vi "Simulated Mecanum Robot.vi"() -> ()   [LabVIEW 2017]
doc: "This example demonstrates the control of an autonomous robot through multiple asynchronous processes, modeled by VIs, that communicate with each other using shared variables. This example also shows an obstacle avoidance algorithm that the simulated robot uses as it navigates. The application includes the following processes:\n\n1. LIDAR Loop (\"Sense\")--Uses LabVIEW dataflow programming to generate simulated sensor data based on the position of the robot and any obstacles in the environment.\n\n2. Operator Loop (\"Think\")--Uses a state machine to control the movement of the robot according to commands from the user. When the robot follows a path without joystick or keyboard control, this process controls the attitude of the autonomous robot using a Vector Field Histogram (VFH) algorithm to avoid obstacles.\n\n3. Motor Loop (\"Act\")--Uses a Control and Simulation Loop, from the Control Design and Simulation Module, to create a model of the robot, simulate its dynamic behavior, and show the control loops and attitude observers."
uses:
  <vilib>/Utility/miscctls.llb/LVPointTypeDef.ctl
  <vilib>/Platform/TimedLoop/XDataNode/timing_clust.ctl
  <vilib>/Platform/TimedLoop/XDataNode/nitl_modes.ctl
  <vilib>/Platform/TimedLoop/XDataNode/wakeup.ctl
  <vilib>/Utility/miscctls.llb/LV3DPointTypeDef.ctl
  <vilib>/Platform/TimedLoop/XDataNode/XDataNode.xnode
  <vilib>/Platform/TimedLoop/XDataNode/XDNodeRunTimeDep.lvlib
panel:
  in  "Show LL Diagram":bool
  in  "Show OL Diagram":bool
  in  "Show MCL Diagram":bool
  out "RR Wheel N":dbl(slide)
  out "RR Wheel":dbl(slide) scale=0.0..15.0
  out "RL Wheel N":dbl(slide)
  out "RL Wheel":dbl(slide) scale=0.0..15.0
  out "FL Wheel N":dbl(slide)
  out "FL Wheel":dbl(slide) scale=0.0..15.0
  out "FR Wheel N":dbl(slide)
  out "FR Wheel":dbl(slide) scale=0.0..15.0
  in  "Rotate Left":dbl(slide) scale=0.0..1.0
  in  "Rotate Right":dbl(slide) scale=0.0..1.0
  in  "Left":dbl(slide)
  in  "Right":dbl(slide) scale=0.0..1.0
  in  "Backward":dbl(slide)
  in  "Forward":dbl(slide) scale=0.0..1.0
  in  "Camera Control":enum32{"Free", "Observer View", "Robot View"}(radio)
  in  "About":bool
  in  "Robot Mode:":enum16{"Idle", "Tele-Op", "Path Following"}(ring)=enum."Tele-Op"
  in  "VFH Visualization":bool
  out "Obstacle Map":picture
  out "End Loop":bool=TRUE
  in  "Stop":bool
  out "3D Visualization":refnum<vi>(3d-picture)
  # "Instructions:\n\n1. If you want to use a joystick to control the simulated robot, install the joystick before you run this VI.\n\n2. Run VI.  Click the About This Example button for more information about the simulated robot.\n\n3. Use the joystick or press keypad buttons to move the robot.\n\n4. Click a position in the Obstacle Map to change the target position of the robot.\n\n5. Click the Robot Mode control and select Path Following to command the robot to navigate to the target based on vector field histogram data about the environment.\n\n6. Click the VFH Visualization button to launch the VFH Visualization VI, in which you can observe the vector field histogram data.\n\n7. Click the buttons in the VI Block Diagram Visualization section to view the code that controls the robot.  You also can press the <Ctrl-E> keys to view the block diagram of the main VI."
  # "VI Block Diagram Visualization"
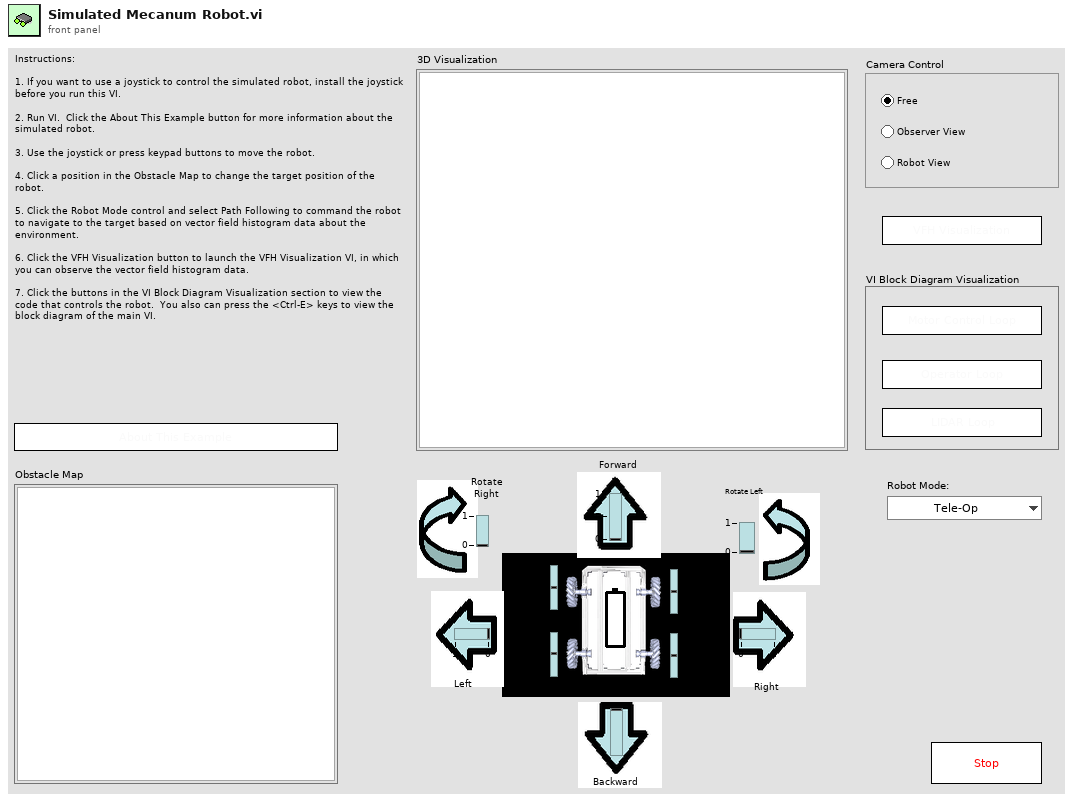
[diagram p1: front panel]
types:
  T1 = typedef "LVPointTypeDef.ctl" = cluster{"Horizontal":i16, "Vertical":i16}
  T2 = typedef "LVBoundsTypeDef.ctl" = cluster{"Width":u32, "Height":u32}
  T3 = typedef "XDNodeRunTimeDep.lvlib/timing_clust.ctl" = cluster{"Expected End [f-1]":u64, "Actual End [f-1]":u64, "Finished Late? [f-1]":bool, "Expected End [i-1]":u64, "Actual End [i-1]":u64, "Finished Late? [i-1]":bool, "Expected Start [i]":u64, "Actual Start [i]":u64, "Expected Start [f]":u64, "Actual Start [f]":u64, "Source Name":string, "Structure Name":string, "Period":i64, "Deadline":i64, "Offset":i64, "Start":i64, "Priority":i32, "Timeout":i32, "Mode":T4, "Wakeup Reason":T5, "Error":errorcluster, "Source Type":string, "Secondary Source Type":string, "Global End Time":u64, "Global Start Time":u64, "Frame Duration":u64, "Iteration Duration":u64, "Assigned CPU":i32, "I/O Scan Engine Mode":u32}
  T4 = typedef "XDNodeRunTimeDep.lvlib/nitl_modes.ctl" = enum32{"No Change", "Process missed periods, maintain original phase", "Discard missed periods, maintain original phase", "Process missed periods, ignore original phase", "Discard missed periods, ignore original phase"}
  T5 = typedef "XDNodeRunTimeDep.lvlib/wakeup.ctl" = enum32{"Normal", "Aborted", "Asynchronous wakeup", "Timing source error", "Timed loop error", "Timeout"}
  T6 = typedef "LVPoint32TypeDef.ctl" = cluster{"Horizontal":i32, "Vertical":i32}
  T7 = typedef "eventvkey.ctl" = enum16{"ASCII", "Enter", "Return", "Shift", "Ctrl", "Alt", "Cmd", "Opt", "Caps", "NumLock", "Clear", "Break", "Up", "Down", "Left", "Right", "Insert", "Delete", "Home", "End", "PageUp", "PageDown", "Escape", "Help", "Pause", "ScrollLock", "F1", "F2", "F3", "F4", "F5", "F6", "F7", "F8", "F9", "F10", "F11", "F12", "F13", "F14", "F15", "F16", "F17", "F18", "F19", "F20", "F21", "F22", "F23", "F24", "Play", "VolumeUp", "VolumeDown", "Mute", "Two Byte Char"}
  T8 = enum16{"Ignore", "Left", "Right", "Up", "Down", "CL", "CC"}
  T9 = typedef "LV3DPointTypeDef.ctl" = cluster{"X":sgl, "Y":sgl, "Z":sgl}
  T10 = cluster{"Array of Double[0]":dbl, "Array of Double[1]":dbl}
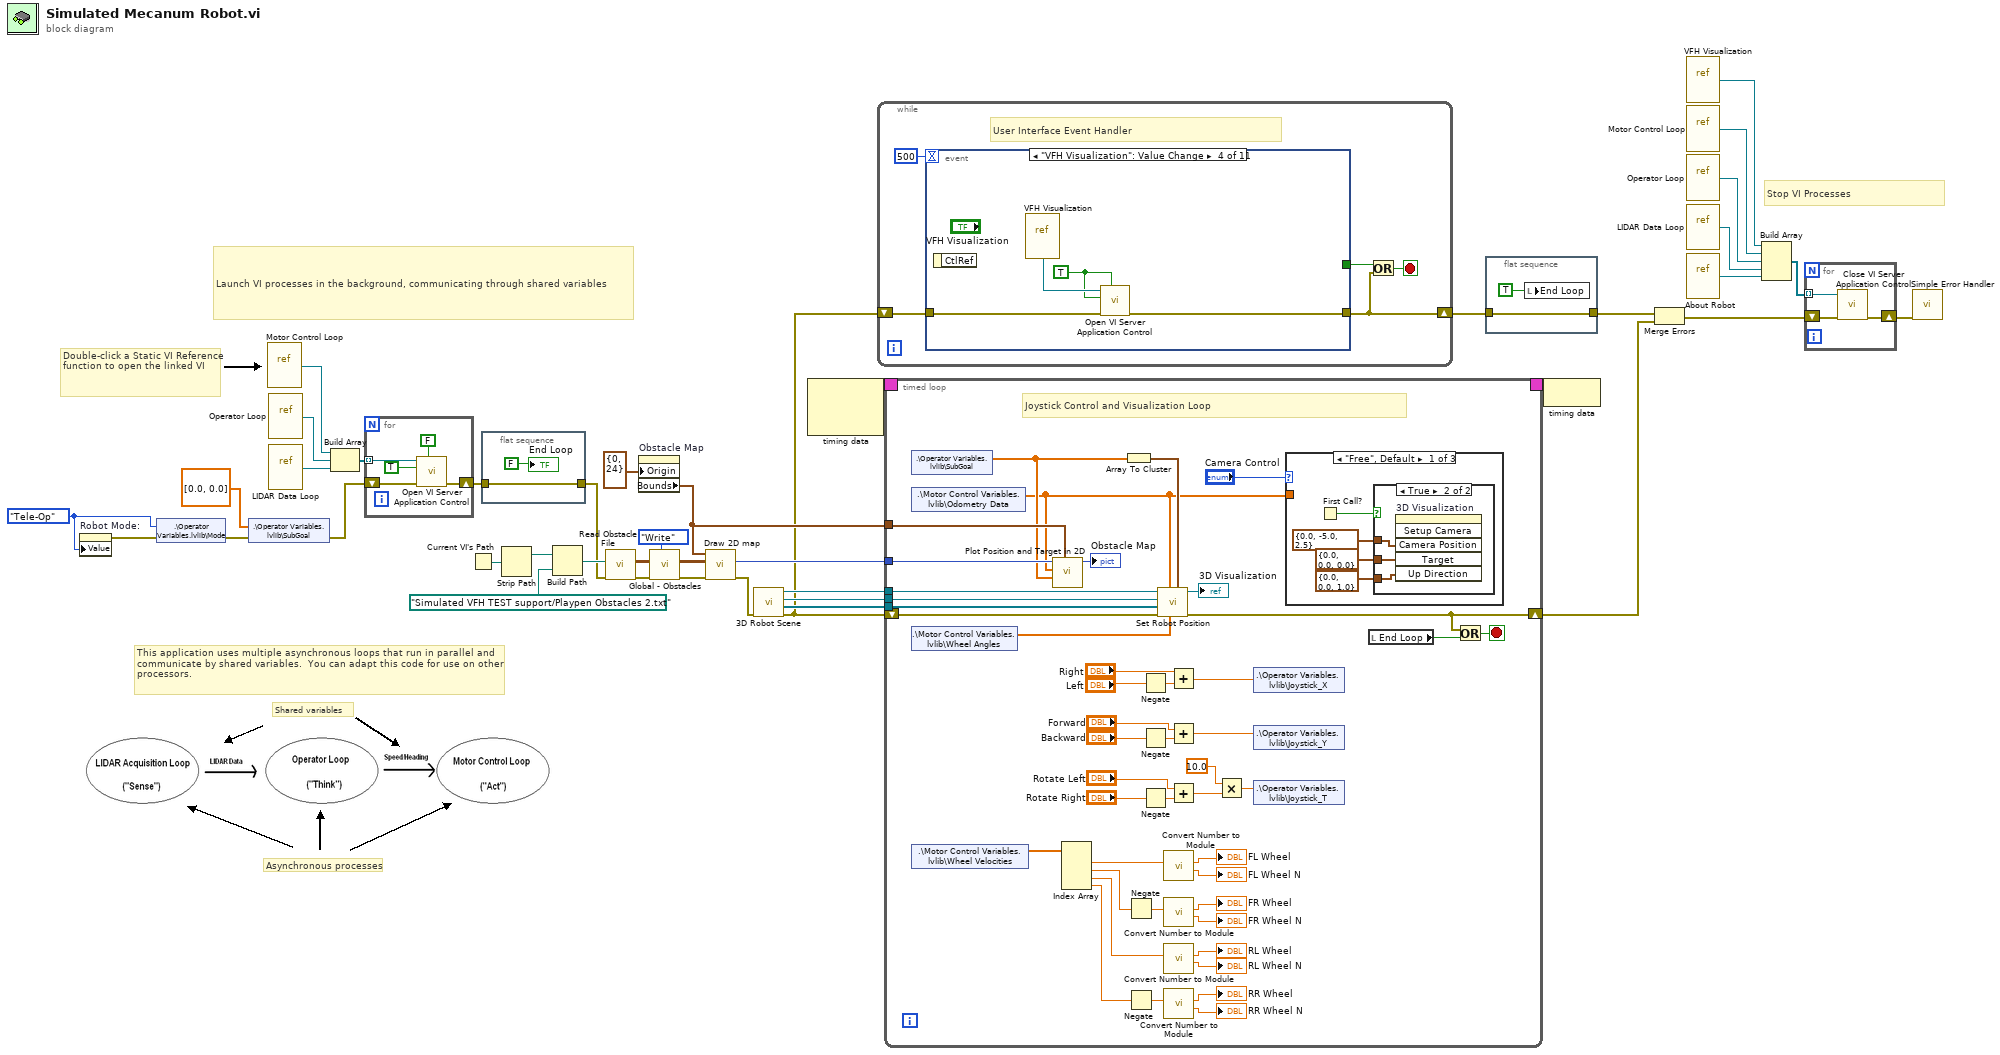
[diagram p0: block diagram]
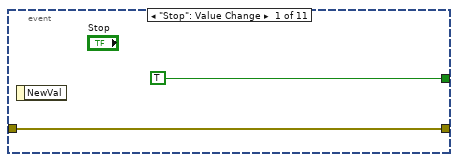
[diagram p2: hidden frame]
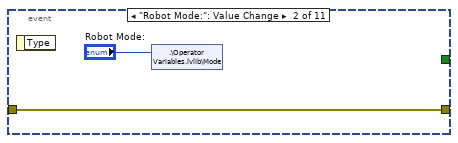
[diagram p3: hidden frame]
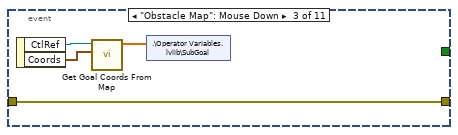
[diagram p4: hidden frame]
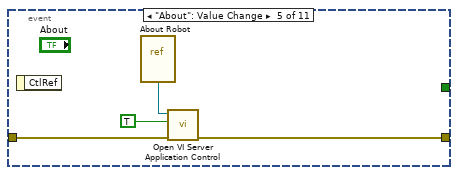
[diagram p5: hidden frame]
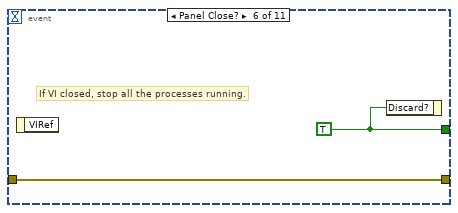
[diagram p6: hidden frame]
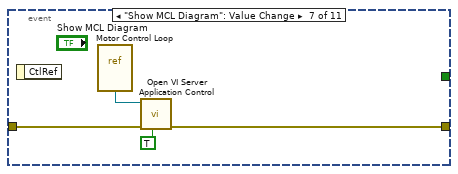
[diagram p7: hidden frame]
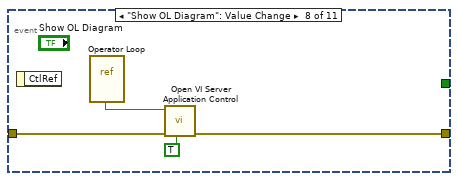
[diagram p8: hidden frame]
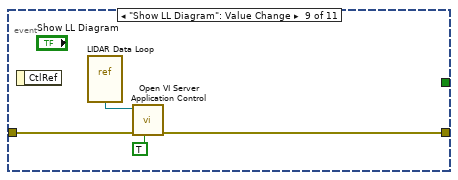
[diagram p9: hidden frame]
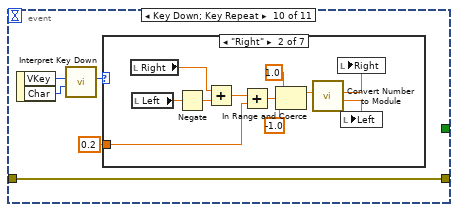
[diagram p10: hidden frame]
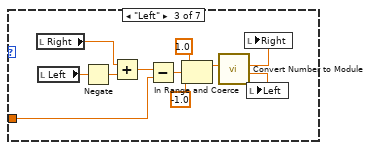
[diagram p12: hidden frame]
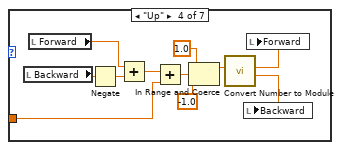
[diagram p13: hidden frame]
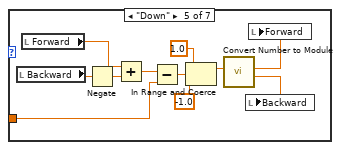
[diagram p14: hidden frame]
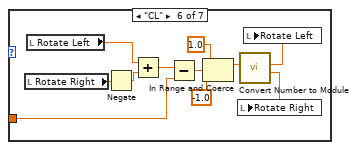
[diagram p15: hidden frame]
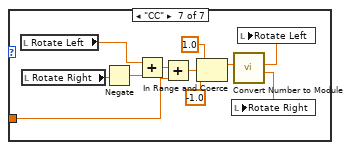
[diagram p16: hidden frame]
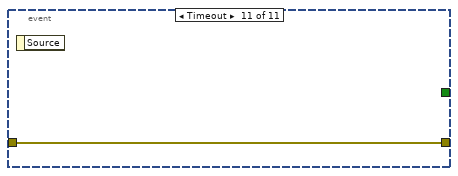
[diagram p17: hidden frame]
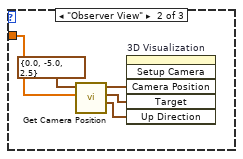
[diagram p19: hidden frame]
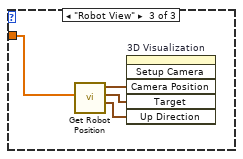
[diagram p20: hidden frame]
diagram:
  w8 = enum16{"Idle", "Tele-Op", "Path Following"}."Tele-Op" ("Mode")
  # "Launch VI processes in the background, communicating through shared variables"
  # "Stop VI Processes"
  # "Shared variables"
  # "Asynchronous processes"
  # "This application uses multiple asynchronous loops that run in parallel and communicate by shared variables.  You can adapt this code for use on other processors."
  # "Double-click a Static VI Reference function to open the linked VI"
  n1 = property on="Robot Mode:" class="Enum (strict)"("Value"=w8) -> (error out=w9:errorcluster)  [unwired: 2 in, 1 out]
  n2 = shared-variable ".\\Operator Variables.lvlib\\Mode"(w8, error in=w9) -> (error out=w4:errorcluster)
  n3 = shared-variable ".\\Operator Variables.lvlib\\SubGoal"(dbl[] [0.0, 0.0] ("SubGoal"), error in=w4) -> (error out=w3:errorcluster)
  n4 = vi-ref "Motor Control Loop.vi"() -> (w26:refnum<vi>)
  n5 = vi-ref "Operator Loop.vi"() -> (w23:refnum<vi>)
  n6 = vi-ref "LIDAR Data Loop.vi"() -> (w22:refnum<vi>)
  n7 = Build Array(w26, w23, w22) -> (w25:refnum<vi>[])
  n8 = for {
    tunnel: w25 -> [w46] mode=indexing
    shift-right: [w43] -> w7
    shift-left: w3 -> [w42]
    n9 = call "Open VI Server Application Control.vi"("open front panel (F)"=FALSE ("Open Front Panel"), "error in (no error)"=w42, "run VI (F)"=TRUE ("Run VI"), "VI refnum"=w46) -> ("error out"=w43:errorcluster)  [unwired: 7 in]
  }
  n10 = Current VI's Path() -> (path=w33:path)
  n11 = flat-sequence {
    tunnel: w7 -> [w48]
    tunnel: [w48] -> w6
    frame #0 {
      "End Loop" <- FALSE ("Halt TL")
    }
  }
  n12 = Strip Path(path=w33) -> (stripped path=w29:path)  [unwired: 1 out]
  n13 = Build Path(base path=w29, name or relative path=path "Simulated VFH TEST support/Playpen Obstacles 2.txt" ("file path for obstacle data")) -> (appended path=w32:path)
  n14 = call "Read Obstacle File.vi"("error in (no error)"=w6, "file path (use dialog)"=w32) -> ("error out"=w34:errorcluster, "obstacles (n x 2 array of pts)"=w35:cluster{dbl, dbl}[][])  [unwired: 8 in]
  n15 = property on="Obstacle Map" class="Pict"("Origin"=T1 {"Horizontal"=0, "Vertical"=24}) -> ("Bounds"=w37:T2)  [unwired: 2 in, 2 out]
  n16 = call "Global - Obstacles.vi"("mode"=enum16{"Initialize", "Read", "Write"}."Write" ("Mode"), "error in (no error)"=w34, "obstacles in"=w35) -> ("error out"=w30:errorcluster, "obstacles out"=w31:cluster{dbl, dbl}[][])  [unwired: 6 in, 1 out]
  n17 = call "Draw 2D map.vi"("error in (no error)"=w30, "obstacles"=w31, "bounds"=w37) -> ("error out"=w24:errorcluster, "picture"=w38:picture)  [unwired: 7 in]
  n18 = call "3D Robot Scene.vi"("error in (no error)"=w24) -> ("error out"=w5:errorcluster, "axles"=w41:refnum<vi>[], "robot"=w40:refnum<vi>, "scene"=w39:refnum<vi>)  [unwired: 7 in]
  n19 = node-c288() -> (w28:T3)  [unwired: 2 in]
  n20 = while {
    shift-right: [w49] -> w13
    shift-left: w5 -> [w53]
    stop <- w52 stop-if-true
    # "User Interface Event Handler"
    n21 = event shown="[3] \"VFH Visualization\": Value Change" {
      selector: _ -> [_ _ _ _ _ _ _ _ _ _ _]
      dyn-events: _ -> [_ _ _ _ _ _ _ _ _ _ _]
      timeout: 500 -> [_ _ _ _ _ _ _ _ _ _ _]
      tunnel: [TRUE _ _ _ _ w70 _ _ _ _ _] -> w51
      tunnel: w53 -> [w55 w56 w58 w63 w68 w71 w73 w77 w81 w84 w155]
      tunnel: [w55 w56 w58 w62 w67 w71 w72 w76 w80 w84 w155] -> w49
      event "Stop": Value Change {
        n22 = event-data() -> ()  [unwired: 2 out]
      }
      event "Robot Mode:": Value Change {
        n23 = event-data() -> ()  [unwired: 2 out]
        n24 = shared-variable ".\\Operator Variables.lvlib\\Mode"("Robot Mode:") -> ()  [unwired: 1 in, 1 out]
      }
      event "Obstacle Map": Mouse Down {
        n25 = event-data() -> ("CtlRef"=w60:refnum<vi>, "Coords"=w59:T6)  [unwired: 1 out]
        n26 = call "Get Goal Coords From Map.vi"("Coords"=w59, "CtlRef"=w60) -> ("Goal Coords"=w61:dbl[])  [unwired: 9 in]
        n27 = shared-variable ".\\Operator Variables.lvlib\\SubGoal"(w61) -> ()  [unwired: 1 in, 1 out]
      }
      event "VFH Visualization": Value Change {
        w64 = TRUE ("Launch Map")
        n28 = event-data() -> ()  [unwired: 2 out]
        n29 = vi-ref "VFH Visualization.vi"() -> (w65:refnum<vi>)
        n30 = call "Open VI Server Application Control.vi"("open front panel (F)"=w64, "error in (no error)"=w63, "run VI (F)"=w64, "VI refnum"=w65) -> ("error out"=w62:errorcluster)  [unwired: 7 in]
      }
      event "About": Value Change {
        n31 = event-data() -> ()  [unwired: 2 out]
        n32 = vi-ref "About Robot.vi"() -> (w69:refnum<vi>)
        n33 = call "Open VI Server Application Control.vi"("error in (no error)"=w68, "run VI (F)"=TRUE ("Launch Map"), "VI refnum"=w69) -> ("error out"=w67:errorcluster)  [unwired: 8 in]
      }
      event Panel Close? {
        w70 = TRUE ("Discard?")
        # "If VI closed, stop all the processes running."
        n34 = event-data() -> ()  [unwired: 2 out]
        n35 = event-data("Discard?"=w70) -> ()  [unwired: 1 in, 1 out]
      }
      event "Show MCL Diagram": Value Change {
        n36 = event-data() -> ()  [unwired: 2 out]
        n37 = vi-ref "Motor Control Loop.vi"() -> (w75:refnum<vi>)
        n38 = call "Open VI Server Application Control.vi"("open block diagram (F)"=TRUE ("Open Front Panel"), "error in (no error)"=w73, "VI refnum"=w75) -> ("error out"=w72:errorcluster)  [unwired: 8 in]
      }
      event "Show OL Diagram": Value Change {
        n39 = event-data() -> ()  [unwired: 2 out]
        n40 = vi-ref "Operator Loop.vi"() -> (w78:refnum<vi>)
        n41 = call "Open VI Server Application Control.vi"("open block diagram (F)"=TRUE ("Open Front Panel"), "error in (no error)"=w77, "VI refnum"=w78) -> ("error out"=w76:errorcluster)  [unwired: 8 in]
      }
      event "Show LL Diagram": Value Change {
        n42 = event-data() -> ()  [unwired: 2 out]
        n43 = vi-ref "LIDAR Data Loop.vi"() -> (w82:refnum<vi>)
        n44 = call "Open VI Server Application Control.vi"("open block diagram (F)"=TRUE ("Open Front Panel"), "error in (no error)"=w81, "VI refnum"=w82) -> ("error out"=w80:errorcluster)  [unwired: 8 in]
      }
      event Key Down; Key Repeat {
        n45 = event-data() -> ("VKey"=w86:T7, "Char"=w87:i16)  [unwired: 1 out]
        n46 = call "Interpret Key Down.vi"("Char"=w87, "VKey"=w86) -> ("Enum"=w85:T8)  [unwired: 9 in]
        n47 = case shown="\"Right\"" w85 {
          tunnel: 0.2 ("y") -> [_ w91 w100 w113 w132 w133 w144]
          frame Default {
          }
          frame "Right" {
            n48 = local read "Right"() -> (w93:dbl)
            n49 = local read "Left"() -> (w92:dbl)
            n50 = Negate(x=w92) -> (-x=w99:dbl)
            n51 = Add(x=w93, y=w99) -> (x+y=w98:dbl)
            n52 = Add(x=w98, y=w91) -> (x+y=w95:dbl)
            n53 = In Range and Coerce(upper limit=1.0, x=w95, lower limit=-1.0) -> (coerced(x)=w94:dbl)  [unwired: 1 out]
            n54 = call "Convert Number to Module.vi"("input"=w94) -> ("Negative Module"=w89:dbl, "Positive Module"=w90:dbl)  [unwired: 9 in]
            n55 = local write "Right"(w90) -> ()
            n56 = local write "Left"(w89) -> ()
          }
          frame "Left" {
            n57 = local read "Right"() -> (w103:dbl)
            n58 = local read "Left"() -> (w104:dbl)
            n59 = Negate(x=w104) -> (-x=w110:dbl)
            n60 = Add(x=w103, y=w110) -> (x+y=w109:dbl)
            n61 = Subtract(x=w109, y=w100) -> (x-y=w106:dbl)
            n62 = In Range and Coerce(upper limit=1.0, x=w106, lower limit=-1.0) -> (coerced(x)=w105:dbl)  [unwired: 1 out]
            n63 = call "Convert Number to Module.vi"("input"=w105) -> ("Negative Module"=w101:dbl, "Positive Module"=w102:dbl)  [unwired: 9 in]
            n64 = local write "Right"(w102) -> ()
            n65 = local write "Left"(w101) -> ()
          }
          frame "Up" {
            n66 = local read "Backward"() -> (w114:dbl)
            n67 = local read "Forward"() -> (w115:dbl)
            n68 = Negate(x=w114) -> (-x=w121:dbl)
            n69 = Add(x=w115, y=w121) -> (x+y=w120:dbl)
            n70 = Add(x=w120, y=w113) -> (x+y=w117:dbl)
            n71 = In Range and Coerce(upper limit=1.0, x=w117, lower limit=-1.0) -> (coerced(x)=w116:dbl)  [unwired: 1 out]
            n72 = call "Convert Number to Module.vi"("input"=w116) -> ("Negative Module"=w111:dbl, "Positive Module"=w112:dbl)  [unwired: 9 in]
            n73 = local write "Backward"(w111) -> ()
            n74 = local write "Forward"(w112) -> ()
          }
          frame "Down" {
            n75 = local read "Backward"() -> (w130:dbl)
            n76 = local read "Forward"() -> (w129:dbl)
            n77 = Negate(x=w130) -> (-x=w131:dbl)
            n78 = Add(x=w129, y=w131) -> (x+y=w128:dbl)
            n79 = Subtract(x=w128, y=w132) -> (x-y=w123:dbl)
            n80 = In Range and Coerce(upper limit=1.0, x=w123, lower limit=-1.0) -> (coerced(x)=w122:dbl)  [unwired: 1 out]
            n81 = call "Convert Number to Module.vi"("input"=w122) -> ("Negative Module"=w126:dbl, "Positive Module"=w127:dbl)  [unwired: 9 in]
            n82 = local write "Backward"(w126) -> ()
            n83 = local write "Forward"(w127) -> ()
          }
          frame "CL" {
            n84 = local read "Rotate Right"() -> (w135:dbl)
            n85 = local read "Rotate Left"() -> (w134:dbl)
            n86 = Negate(x=w135) -> (-x=w143:dbl)
            n87 = Add(x=w134, y=w143) -> (x+y=w142:dbl)
            n88 = Subtract(x=w142, y=w133) -> (x-y=w139:dbl)
            n89 = In Range and Coerce(upper limit=1.0, x=w139, lower limit=-1.0) -> (coerced(x)=w138:dbl)  [unwired: 1 out]
            n90 = call "Convert Number to Module.vi"("input"=w138) -> ("Negative Module"=w136:dbl, "Positive Module"=w137:dbl)  [unwired: 9 in]
            n91 = local write "Rotate Right"(w136) -> ()
            n92 = local write "Rotate Left"(w137) -> ()
          }
          frame "CC" {
            n93 = local read "Rotate Left"() -> (w145:dbl)
            n94 = local read "Rotate Right"() -> (w146:dbl)
            n95 = Negate(x=w146) -> (-x=w153:dbl)
            n96 = Add(x=w145, y=w153) -> (x+y=w152:dbl)
            n97 = Add(x=w152, y=w144) -> (x+y=w149:dbl)
            n98 = In Range and Coerce(upper limit=1.0, x=w149, lower limit=-1.0) -> (coerced(x)=w148:dbl)  [unwired: 1 out]
            n99 = call "Convert Number to Module.vi"("input"=w148) -> ("Negative Module"=w147:dbl, "Positive Module"=w154:dbl)  [unwired: 9 in]
            n100 = local write "Rotate Right"(w147) -> ()
            n101 = local write "Rotate Left"(w154) -> ()
          }
        }
      }
      event Timeout {
        n102 = event-data() -> ()  [unwired: 2 out]
      }
    }
    n103 = Or(x=w51, y=w49) -> (x .or. y?=w52:bool)
  }
  n104 = timed-loop {
    timing: w28 -> [_]
    timing-out: [_] -> w27
    tunnel: w39 -> [w191]
    tunnel: w40 -> [w190]
    tunnel: w41 -> [w189]
    tunnel: w38 -> [w196]
    tunnel: w37 -> [w194]
    shift-right: [w156] -> w10
    shift-left: w5 -> [w176]
    stop <- w174 stop-if-true
    # "Joystick Control and Visualization Loop"
    n105 = shared-variable ".\\Operator Variables.lvlib\\SubGoal"() -> (w193:dbl[])  [unwired: 1 in, 1 out]
    n106 = shared-variable ".\\Motor Control Variables.lvlib\\Odometry Data"() -> (w177:dbl[])  [unwired: 1 in, 1 out]
    n107 = shared-variable ".\\Motor Control Variables.lvlib\\Wheel Angles"() -> (w188:dbl[])  [unwired: 1 in, 1 out]
    n108 = shared-variable ".\\Motor Control Variables.lvlib\\Wheel Velocities"() -> (w186:dbl[])  [unwired: 1 in, 1 out]
    n109 = call "Plot Position and Target in 2D.vi"("bounds"=w194, "sub-goal"=w193, "odometry data"=w177, "picture in"=w196) -> ("picture out"=→"Obstacle Map":picture)  [unwired: 7 in]
    n110 = Index Array(array=w186) -> (element #1=w173:dbl, element #2=w172:dbl, element #3=w170:dbl, element #4=w169:dbl)  [unwired: 4 in]
    n111 = Array To Cluster(array=w193) -> (cluster=w192:T10)
    n112 = Negate(x=w172) -> (-x=w171:dbl)
    n113 = Negate(x=w169) -> (-x=w168:dbl)
    n114 = Negate(x="Left") -> (-x=w164:dbl)
    n115 = Negate(x="Backward") -> (-x=w167:dbl)
    n116 = Negate(x="Rotate Right") -> (-x=w163:dbl)
    n117 = call "Set Robot Position.vi"("Goal"=w192, "Wheel theta"=w188, "Odometry Data"=w177, "error in (no error)"=w176, "axles"=w189, "robot"=w190, "scene in"=w191) -> ("error out"=w156:errorcluster, "scene out"=→"3D Visualization":refnum<vi>)  [unwired: 3 in]
    n118 = call "Convert Number to Module.vi"("input"=w173) -> ("Negative Module"=→"FL Wheel N":dbl, "Positive Module"=→"FL Wheel":dbl)  [unwired: 9 in]
    n119 = call "Convert Number to Module.vi"("input"=w171) -> ("Negative Module"=→"FR Wheel N":dbl, "Positive Module"=→"FR Wheel":dbl)  [unwired: 9 in]
    n120 = call "Convert Number to Module.vi"("input"=w170) -> ("Negative Module"=→"RL Wheel N":dbl, "Positive Module"=→"RL Wheel":dbl)  [unwired: 9 in]
    n121 = call "Convert Number to Module.vi"("input"=w168) -> ("Negative Module"=→"RR Wheel N":dbl, "Positive Module"=→"RR Wheel":dbl)  [unwired: 9 in]
    n122 = Add(x="Right", y=w164) -> (x+y=w199:dbl)
    n123 = Add(x="Forward", y=w167) -> (x+y=w198:dbl)
    n124 = Add(x="Rotate Left", y=w163) -> (x+y=w160:dbl)
    n125 = Multiply(x=10.0, y=w160) -> (x*y=w197:dbl)
    n126 = shared-variable ".\\Operator Variables.lvlib\\Joystick_X"(w199) -> ()  [unwired: 1 in, 1 out]
    n127 = shared-variable ".\\Operator Variables.lvlib\\Joystick_Y"(w198) -> ()  [unwired: 1 in, 1 out]
    n128 = shared-variable ".\\Operator Variables.lvlib\\Joystick_T"(w197) -> ()  [unwired: 1 in, 1 out]
    n129 = case shown="\"Free\", Default" "Camera Control" {
      tunnel: w177 -> [_ w211 w213]
      frame "Free", Default {
        n130 = First Call?() -> (First Call?: T/F=w204:bool)
        n131 = case shown="True" w204 {
          tunnel: T9 {"X"=0.0, "Y"=-5.0, "Z"=2.5} ("Camera Position") -> [_ w207]
          tunnel: T9 {"X"=0.0, "Y"=0.0, "Z"=0.0} ("Target") -> [_ w206]
          tunnel: T9 {"X"=0.0, "Y"=0.0, "Z"=1.0} ("Up Direction") -> [_ w205]
          frame False {
          }
          frame True {
            n132 = invoke on="3D Visualization" class="SceneGraphDisp (strict)" method="Setup Camera"("Camera Position"=w207, "Target"=w206, "Up Direction"=w205) -> ()  [unwired: 3 in, 6 out]
          }
        }
      }
      frame "Observer View" {
        n133 = call "Get Camera Position.vi"("Odometry Data"=w211, "Camera Position"=T9 {"X"=0.0, "Y"=-5.0, "Z"=2.5}) -> ("Up Direction"=w209:cluster{"index":sgl, "index":sgl, "index":sgl}, "Target"=w210:cluster{"DBL":dbl, "DBL":dbl, "index":sgl}, "Camera Position"=w212:cluster{dbl, dbl, sgl})  [unwired: 7 in]
        n134 = invoke on="3D Visualization" class="SceneGraphDisp (strict)" method="Setup Camera"("Camera Position"=w212, "Target"=w210, "Up Direction"=w209) -> ()  [unwired: 3 in, 6 out]
      }
      frame "Robot View" {
        n135 = call "Get Robot Position.vi"("Odometry Data"=w213) -> ("Up Direction"=w214:cluster{"index":sgl, "index":sgl, "index":sgl}, "Target"=w215:cluster{"DBL":dbl, "DBL":dbl, "index":sgl}, "Camera Position"=w216:cluster{dbl, dbl, sgl})  [unwired: 8 in]
        n136 = invoke on="3D Visualization" class="SceneGraphDisp (strict)" method="Setup Camera"("Camera Position"=w216, "Target"=w215, "Up Direction"=w214) -> ()  [unwired: 3 in, 6 out]
      }
    }
    n137 = local read "End Loop"() -> (w175:bool)
    n138 = Or(x=w156, y=w175) -> (x .or. y?=w174:bool)
  }
  n139 = flat-sequence {
    tunnel: w13 -> [w220]
    tunnel: [w220] -> w12
    frame #0 {
      n140 = local write "End Loop"(TRUE ("End Loop")) -> ()
    }
  }
  n141 = node-c288(w27) -> ()
  n142 = Merge Errors(w12, w10) -> (w11:errorcluster)
  n143 = vi-ref "VFH Visualization.vi"() -> (w16:refnum<vi>)
  n144 = vi-ref "Motor Control Loop.vi"() -> (w20:refnum<vi>)
  n145 = vi-ref "Operator Loop.vi"() -> (w19:refnum<vi>)
  n146 = vi-ref "LIDAR Data Loop.vi"() -> (w18:refnum<vi>)
  n147 = vi-ref "About Robot.vi"() -> (w15:refnum<vi>)
  n148 = Build Array(w16, w20, w19, w18, w15) -> (w17:refnum<vi>[])
  n149 = for {
    tunnel: w17 -> [w223] mode=indexing
    shift-right: [w222] -> w14
    shift-left: w11 -> [w221]
    n150 = call "Close VI Server Application Control.vi"("error in (no error)"=w221, "VI refnum"=w223) -> ("error out"=w222:errorcluster)  [unwired: 9 in]
  }
  n151 = call <vilib>:"Simple Error Handler.vi"("error in (no error)"=w14) -> ()  [unwired: 4 in, 5 out]
